vi "EMV Check For Decreasing Temperatures.vi"(8 "error in (no error)":errorcluster, 11 "Current T7 Temperatures":dbl[](array[numeric])) -> (0 "error out":errorcluster, 2 "Slope History":dbl[](array[numeric]), 3 "Current T7 Temperatures Output":dbl[](array[numeric]), 5 "Detection?":bool)   [LabVIEW 2016]
uses:
  <vilib>/Analysis/baseanly.llb/Mean (DBL).vi
  <vilib>/Analysis/NI_AALBase.lvlib
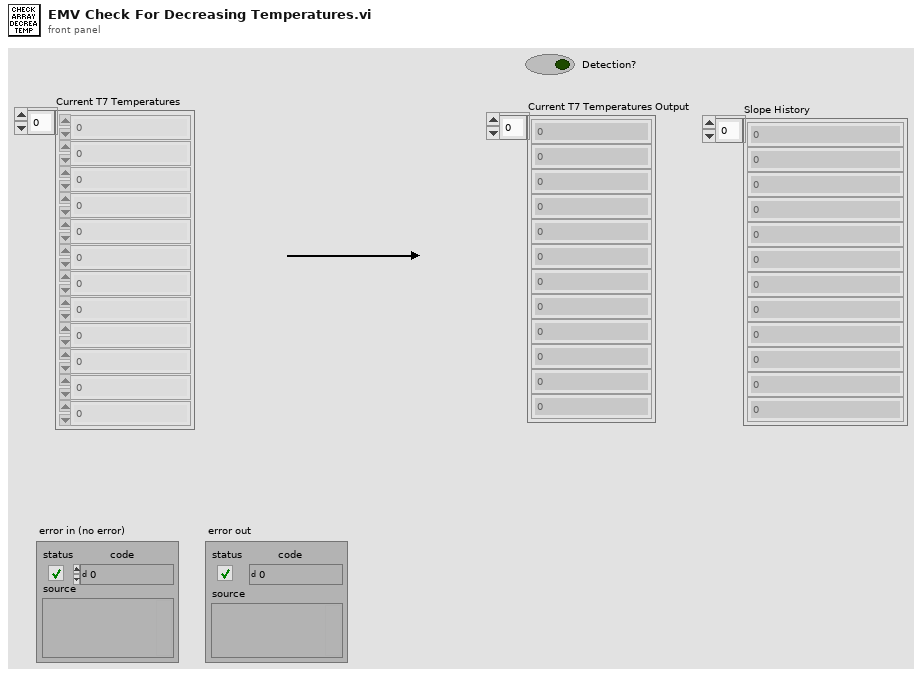
[diagram p1: front panel]
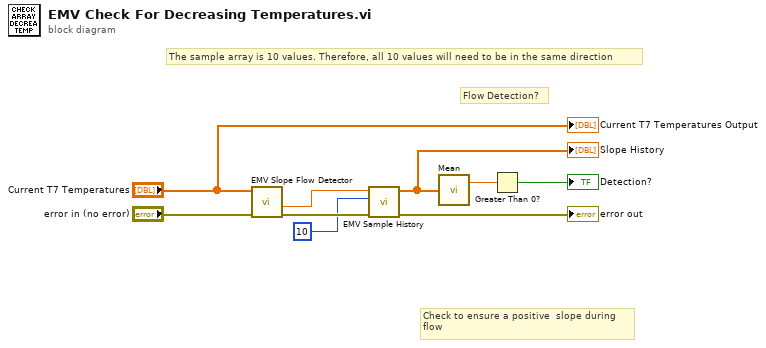
[diagram p0: block diagram]
diagram:
  # "Flow Detection?"
  # "Check to ensure a positive  slope during\nflow"
  # "The sample array is 10 values. Therefore, all 10 values will need to be in the same direction"
  n1 = call "EMV Slope Flow Detector.vi"("error in (no error)"="error in (no error)", "Current T6 Temperatures in"="Current T7 Temperatures") -> ("error out"=w9:errorcluster, "slope"=w8:dbl)  [unwired: 7 in, 1 out]
  n2 = call "EMV Sample History.vi"("error in (no error)"=w9, "length"=10, "T6 Temp"=w8) -> ("error out"=→"error out":errorcluster, "T6 History"=w5:dbl[])  [unwired: 7 in]
  "Slope History" <- w5
  n3 = call-poly <vilib>:"Mean.vi"("X"=w5) -> ("mean"=w4:dbl)  [unwired: 1 out]
  n4 = Greater Than 0?(x=w4) -> (x > 0?=→"Detection?":bool)
  "Current T7 Temperatures Output" <- "Current T7 Temperatures"
